vi "LoopselFFcont.VI"() -> ()   [LabVIEW 2015]
panel:
  in  "?":enum32{"1", "2", "3"}(radio)=enum."3"
  in  "pos slope":u8=1
  in  "both slopes":u8
  in  "DAT in 10ns":u32
  out "FIFO overflow":bool
  in  "extTrig 0/1":u8
  in  "stop all":bool
  in  "Slide":u32(slide)=43 scale=1.0..100.0
  in  "frequency[Hz]":u32
  in  "no.of samples (nos)":u32=100
  in  "exposuretime[ms]":dbl=1.0 format="%.3f"
  out "Signalverlaufgraph":u16[](graph)=[4076, 4076, 4076, 4076, 49152, 0, 42, 0, 5277, 5276, 5280, 5289, 5299, 5320, 5298, 5313, 5292, 5320, 5318, 5328, 5333, 5340, 5328, 5331, 5343, 5348, 5338, 5328, 5328, 5329, 5336, 5335, 5343, 5341, 5341, 5331, 5348, 5353, 5349, 5352, 5361, 5365, 5360, 5360, 5367, 5365, 5362, 5372, 5378, 5366, 5379, 5376, 5365, 5378, 5379, 5391, 5376, 5374, 5392, 5411, 5401, 5385, 5382, 5389, 5397, 5390, 5364, 5369, 5381, 5387, 5391, 5387, 5376, 5398, 5395, 5387, 5382, 5377, 5391, 5398, 5407, 5399, 5401, 5418, 5398, 5400, 5391, 5404, 5396, 5394, 5397, 5401, 5390, 5402, 5392, 5394, 5393, 5388, 5389, 5398, 5391, 5377, 5375, 5369, 5388, 5357, 5365, 5359, 5339, 5362, 5354, 5366, 5361, 5352, 5356, 5360, 5352, 5361, 5380, 5378, 5373, 5373, 5365, 5374, 5354, 5364, 5360, 5369, 5367, 5378, 5367, 5382, 5379, 5375, 5378, 5378, 5370, 5369, 5369, 5356, 5359, 5383, 5364, 5356, 5342, 5368, 5376, 5359, 5360, 5367, 5363, 5361, 5379, 5390, 5374, 5346, 5368, 5351, 5390, 5373, 5387, 5363, 5350, 5351, 5347, 5345, 5334, 5331, 5350, 5320, 5328, 5341, 5326, 5327, 5342, 5334, 5340, 5335, 5338, 5335, 5343, 5340, 5337, 5359, 5339, 5331, 5336, 5360, 5345, 5329, 5333, 5327, 5332, 5330, 5309, 5327, 5328, 5332, 5342, 5313, 5304, 5334, 5322, 5319, 5315, 5297, 5310, 5310, 5310, 5293, 5295, 5311, 5285, 5296, 5281, 5297, 5277, 5279, 5293, 5288, 5281, 5286, 5278, 5275, 5273, 5289, 5286, 5283, 5297, 5266, 5268, 5273, 5283, 5269, 5278, 5270, 5268, 5276, 5274, 5272, 5259, 5279, 5263, 5268, 5244, 5265, 5278, 5267, 5259, 5252, 5265, 5266, 5246, 5255, 5257, 5252, 5259, 5274, 5268, 5292, 5296, 5291, 5292, 5292, 5310, 5310, 5324, 5316, 5321, 5344, 5332, 5325, 5305, 5339, 5336, 5340, 5329, 5337, 5345, 5341, 5354, 5368, 5352, 5334, 5347, 5344, 5372, 5364, 5377, 5385, 5370, 5350, 5380, 5375, 5378, 5362, 5379, 5359, 5363, 5365, 5363, 5365, 5357, 5354, 5358, 5342, 5371, 5380, 5370, 5382, 5376, 5399, 5377, 5365, 5370, 5386, 5389, 5360, 5380, 5387, 5364, 5379, 5363, 5363, 5382, 5378, 5390, 5364, 5347, 5386, 5379, 5372, 5361, 5371, 5386, 5386, 5402, 5393, 5402, 5415, 5400, 5411, 5393, 5410, 5402, 5403, 5408, 5412, 5402, 5394, 5396, 5388, 5381, 5387, 5407, 5378, 5384, 5369, 5393, 5386, 5397, 5394, 5393, 5377, 5392, 5391, 5406, 5397, 5389, 5395, 5387, 5391, 5379, 5384, 5397, 5412, 5397, 5395, 5393, 5388, 5368, 5391, 5392, 5391, 5401, 5399, 5396, 5407, 5407, 5395, 5392, 5392, 5433, 5425, 5438, 5441, 5446, 5473, 5438, 5453, 5424, 5444, 5449, 5459, 5448, 5468, 5474, 5465, 5488, 5502, 5495, 5473, 5482, 5483, 5500, 5503, 5509, 5508, 5502, 5496, 5520, 5515, 5518, 5521, 5517, 5515, 5534, 5527, 5538, 5546, 5539, 5543, 5546, 5543, 5572, 5561, 5569, 5565, 5563, 5590, 5572, 5574, 5561, 5583, 5582, 5555, 5556, 5559, 5547, 5558, 5543, 5542, 5558, 5560, 5581, 5561, 5558, 5571, 5565, 5561, 5564, 5554, 5572, 5585, 5590, 5579, 5597, 5609, 5602, 5601, 5606, 5627, 5597, 5630, 5632, 5640, 5622, 5635, 5634, 5641, 5632, 5622, 5640, 5637, 5624, 5586, 5615, 5619, 5629, 5611, 5612, 5595, 5603, 5614, 5615, 5613, 5608, 5624, 5626, 5642, 5635, 5653, 5677, 5682, 5697, 5701, 5696, 5712, 5691, 5709, 5699, 5708, 5725, 5733, 5722, 5737, 5734, 5716, 5723, 5723, 5737, 5730, 5731, 5736, 5752, 5763, 5751, 5762, 5722, 5747, 5753, 5752, 5761, 5766, 5764, 5767, 5778, 5808, 5801, 5781, 5795, 5789, 5812, 5816, 5834, 5823, 5815, 5817, 5848, 5831, 5831, 5827, 5848, 5827, 5840, 5831, 5852, 5852, 5850, 5840, 5842, 5845, 5867, 5858, 5848, 5840, 5851, 5866, 5834, 5847, 5847, 5884, 5865, 5841, 5855, 5847, 5857, 5850, 5844, 5843, 5867, 5848, 5871, 5849, 5845, 5873, 5860, 5844, 5845, 5838, 5852, 5846, 5853, 5841, 5861, 5862, 5859, 5847, 5825, 5845, 5821, 5813, 5807, 5814, 5793, 5801, 5775, 5768, 5752, 5755, 5778, 5751, 5756, 5726, 5745, 5747, 5760, 5742, 5755, 5727, 5712, 5745, 5731, 5726, 5704, 5715, 5707, 5712, 5697, 5688, 5697, 5705, 5707, 5685, 5681, 5685, 5664, 5685, 5674, 5683, 5676, 5684, 5670, 5687, 5680, 5704, 5678, 5678, 5660, 5673, 5685, 5664, 5684, 5718, 5688, 5685, 5682, 5716, 5712, 5713, 5733, 5734, 5731, 5736, 5750, 5765, 5760, 5754, 5768, 5761, 5794, 5804, 5808, 5817, 5813, 5797, 5829, 5806, 5809, 5824, 5835, 5823, 5833, 5821, 5843, 5845, 5848, 5847, 5846, 5828, 5855, 5847, 5860, 5860, 5858, 5861, 5847, 5847, 5841, 5865, 5876, 5844, 5852, 5873, 5879, 5888, 5869, 5884, 5895, 5908, 5918, 5915, 5886, 5942, 5943, 5932, 5935, 5932, 5977, 5963, 5976, 5979, 5979, 5999, 5986, 6002, 6013, 6019, 6011, 6022, 6029, 6053, 6040, 6062, 6043, 6065, 6060, 6070, 6095, 6094, 6091, 6075, 6091, 6109, 6134, 6116, 6119, 6126, 6145, 6168, 6166, 6189, 6187, 6202, 6192, 6203, 6201, 6197, 6236, 6232, 6250, 6238, 6240, 6258, 6248, 6298, 6256, 6278, 6284, 6321, 6320, 6347, 6357, 6341, 6345, 6345, 6484, 6493, 6520, 6543, 6543, 6596, 6575, 6598, 6565, 6617, 6650, 6652, 6654, 6659, 6702, 6704, 6716, 6734, 6744, 6707, 6760, 6758, 6785, 6797, 6825, 6851, 6833, 6859, 6862, 6902, 6909, 6930, 6946, 6957, 6966, 7001, 7009, 7030, 7060, 7051, 7095, 7116, 7137, 7180, 7173, 7176, 7226, 7247, 7272, 7282, 7297, 7337, 7352, 7357, 7385, 7400, 7423, 7458, 7457, 7494, 7517, 7522, 7573, 7573, 7598, 7628, 7654, 7677, 7699, 7709, 7743, 7781, 7792, 7806, 7833, 7861, 7890, 7918, 7938, 7975, 8007, 8039, 8071, 8201, 8343, 8472, 8545, 8684, 8781, 8900, 9041, 9174, 9328, 9463, 9699, 9865, 9976, 10092, 10188, 10266, 10363, 10476, 10562, 10647, 10724, 10818, 10899, 10992, 11048, 11133, 11209, 11299, 11364, 11432, 11512, 11636, 11765, 11921, 12014, 11754, 12235, 12262, 12168, 12214, 12077, 12308, 11568, 11568, 12560, 12073, 12414, 11719, 12059, 12077, 12213, 12350, 12026, 12183, 11918, 11864, 12055, 12342, 12128, 11867, 12416, 12025, 12192, 11997, 12278, 11898, 12191, 12431, 12115, 12141, 11903, 12153, 12110, 11801, 12437, 12528, 12423, 11932, 12627, 12345, 12149, 12615, 12257, 12116, 12293, 11953, 12603, 12261, 12666, 12662, 12225, 12318, 12508, 12002, 12565, 12622, 12199, 12454, 12372, 12103, 12123, 12331, 12088, 12322, 12482, 12010, 12523, 12404, 12269, 12063, 12353, 11857, 12358, 12007, 12339, 12372, 12229, 12499, 12305, 12533, 12477, 12282, 11918, 12526, 12075, 12314, 12043, 12445, 11842, 12154, 11837, 12170, 13169, 12522, 13214, 12892, 12475, 12217, 12608, 12192, 12477, 12321, 12296, 12480, 12396, 12554, 12225, 12268, 12325, 11818, 12342, 12080, 12362, 12168, 12424, 11750, 12150, 12974, 12289, 12219, 12437, 12227, 12272, 12068, 12123, 11755, 12117, 11840, 11624, 12420, 12486, 12486, 4083, 4084, 4104, 4092, 4088, 4082, 4083, 4082, 4086, 4086, 4081, 4096, 4095, 4082, 4084, 4086, 4081, 4088, 4067, 4081, 4078, 4080, 4088, 4088, 4086, 4080, 4092, 4080, 4078, 4082, 4082, 4082, 4097, 4099, 4099, 4093, 4079, 4092, 4082, 4087, 4086, 4088, 4091, 4085, 4088, 4084, 4086, 4091, 4091, 4079, 4078, 4090, 4095, 4095, 4095, 4095]
  # "Start with run"
  # "Abort with ESC"
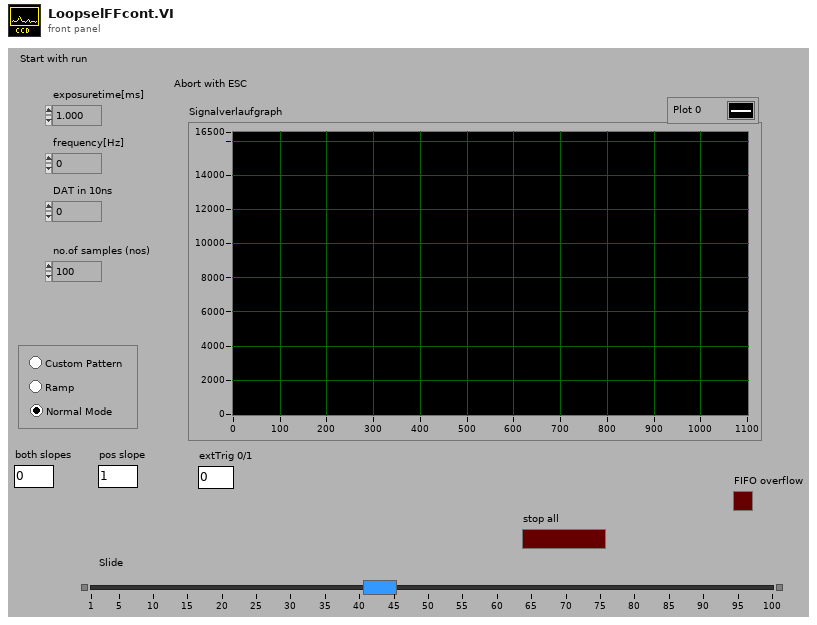
[diagram p1: front panel]
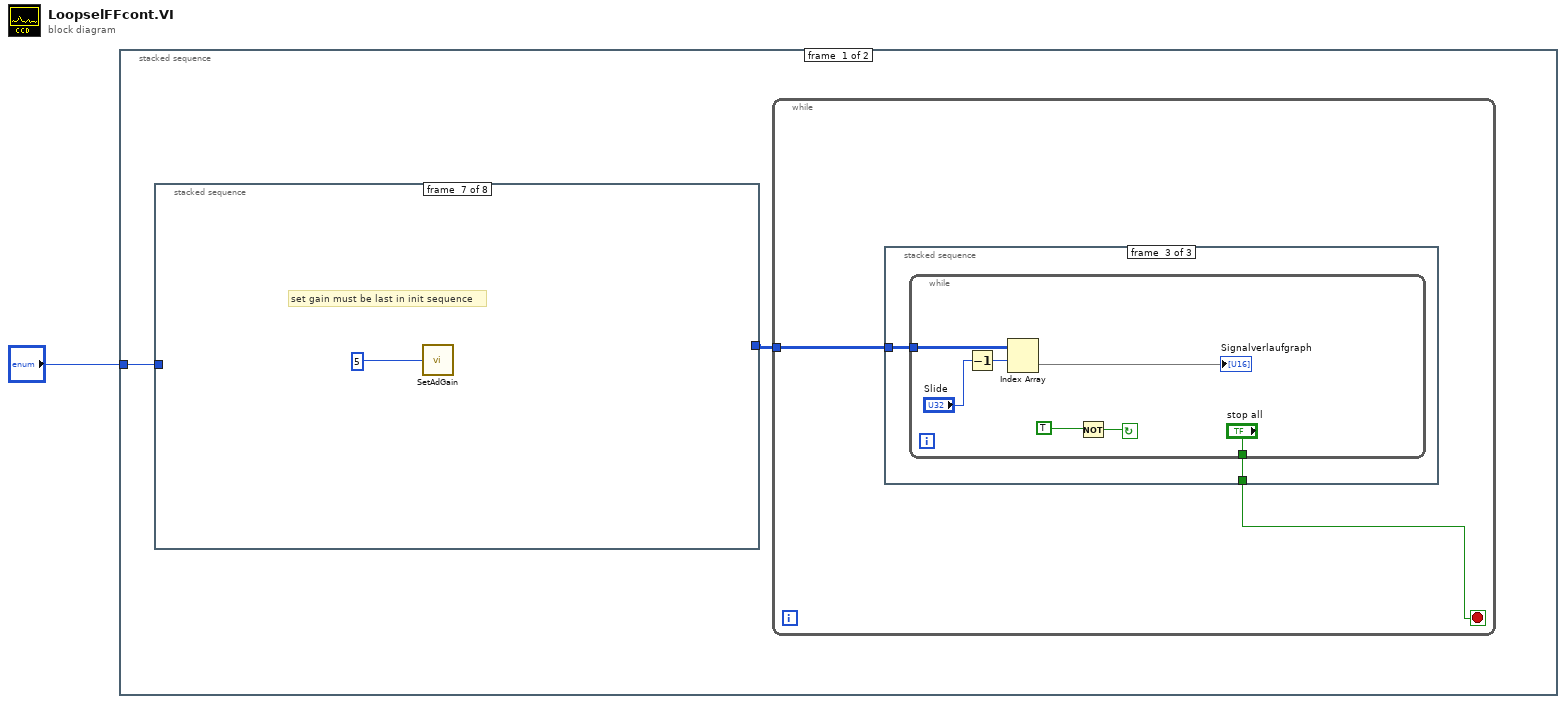
[diagram p0: block diagram]
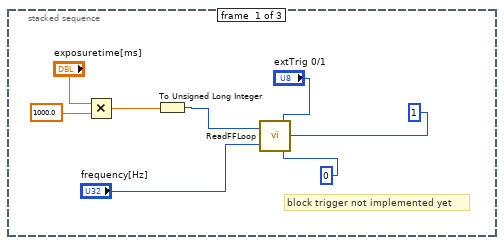
[diagram p2: hidden frame]
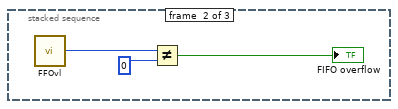
[diagram p3: hidden frame]
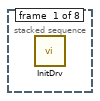
[diagram p4: hidden frame]
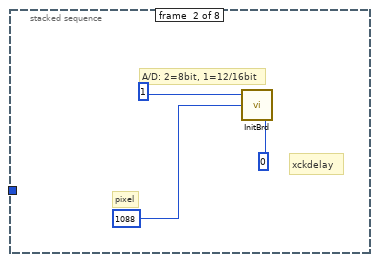
[diagram p5: hidden frame]
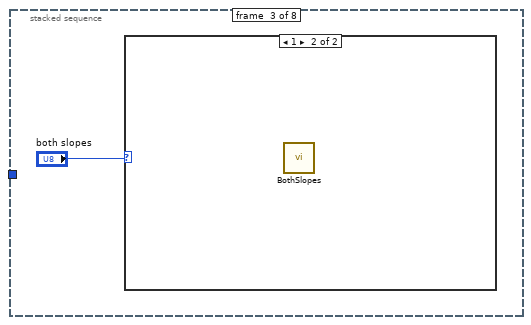
[diagram p6: hidden frame]
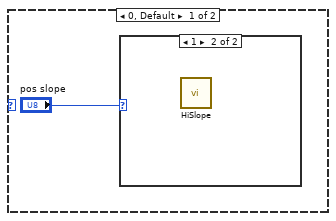
[diagram p7: hidden frame]
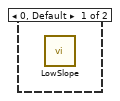
[diagram p8: hidden frame]
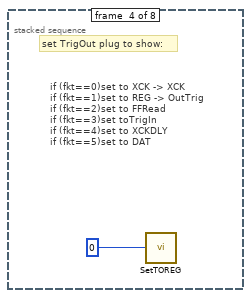
[diagram p9: hidden frame]
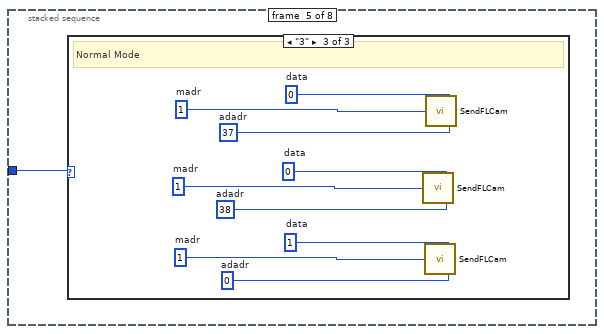
[diagram p10: hidden frame]
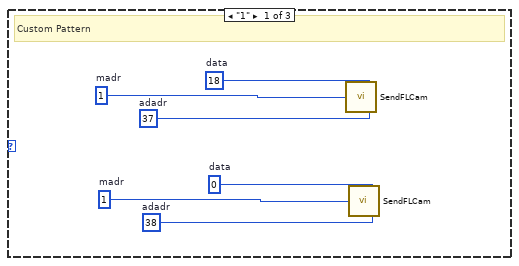
[diagram p11: hidden frame]
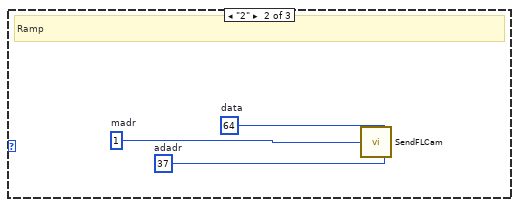
[diagram p12: hidden frame]
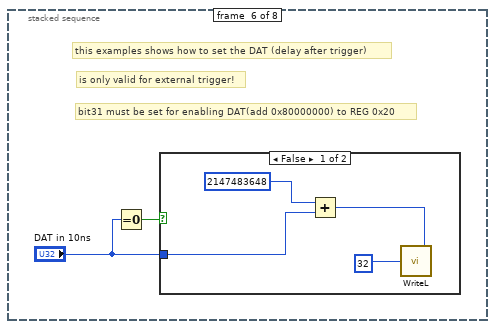
[diagram p13: hidden frame]
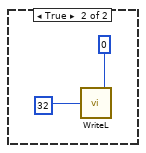
[diagram p14: hidden frame]
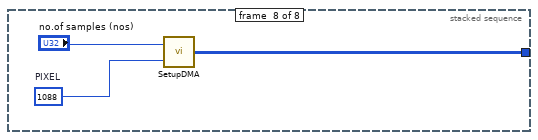
[diagram p15: hidden frame]
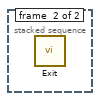
[diagram p16: hidden frame]
diagram:
  n1 = stacked-sequence {
    tunnel: "?" -> [w2 _]
    frame #0 {
      n2 = stacked-sequence {
        tunnel: [_ _ _ _ _ _ _ w62] -> w3
        tunnel: w2 -> [_ _ _ _ w32 _ _ _]
        frame #0 {
          n3 = call "InitDrv.vi"() -> ()  [unwired: 1 in]
        }
        frame #1 {
          # "pixel"
          # "xckdelay"
          # "A/D: 2=8bit, 1=12/16bit"
          n4 = call "InitBrd.vi"("xckdly"=u32 0, "pixel"=u32 1088, "flag816"=u32 1) -> ()  [unwired: 3 in]
        }
        frame #2 {
          n5 = case shown="1" "both slopes" {
            frame 0, Default {
              n6 = case shown="1" "pos slope" {
                frame 0, Default {
                  n7 = call "LowSlope.vi"() -> ()  [unwired: 1 in]
                }
                frame 1 {
                  n8 = call "HiSlope.vi"() -> ()  [unwired: 1 in]
                }
              }
            }
            frame 1 {
              n9 = call "BothSlopes.vi"() -> ()  [unwired: 1 in]
            }
          }
        }
        frame #3 {
          # "set TrigOut plug to show:"
          # "if (fkt==0)set to XCK -> XCK\nif (fkt==1)set to REG -> OutTrig\nif (fkt==2)set to FFRead\nif (fkt==3)set toTrigIn\nif (fkt==4)set to XCKDLY\nif (fkt==5)set to DAT"
          n10 = call "SetTOREG.vi"("fkt"=u8 0) -> ()
        }
        frame #4 {
          n11 = case shown="\"3\"" w32 {
            frame "1" {
              w33 = 0  # data
              w34 = 38  # adadr
              w35 = 1  # madr
              w36 = 18  # data
              w37 = 37  # adadr
              w38 = 1  # madr
              # "Custom Pattern"
              n12 = call "SendFLCam.vi"("madr"=w38, "data"=w36, "adadr"=w37) -> ()
              n13 = call "SendFLCam.vi"("madr"=w35, "data"=w33, "adadr"=w34) -> ()
            }
            frame "2" {
              w39 = 64  # data
              w40 = 37  # adadr
              w41 = 1  # madr
              # "Ramp"
              n14 = call "SendFLCam.vi"("madr"=w41, "data"=w39, "adadr"=w40) -> ()
            }
            frame "3" {
              w42 = 1  # data
              w44 = 0  # adadr
              w43 = 1  # madr
              w47 = 0  # data
              w46 = 38  # adadr
              w45 = 1  # madr
              w50 = 0  # data
              w49 = 37  # adadr
              w48 = 1  # madr
              # "Normal Mode"
              n15 = call "SendFLCam.vi"("madr"=w45, "data"=w47, "adadr"=w46) -> ()
              n16 = call "SendFLCam.vi"("madr"=w43, "data"=w42, "adadr"=w44) -> ()
              n17 = call "SendFLCam.vi"("madr"=w48, "data"=w50, "adadr"=w49) -> ()
            }
          }
        }
        frame #5 {
          # "bit31 must be set for enabling DAT(add 0x80000000) to REG 0x20"
          # "is only valid for external trigger!"
          # "this examples shows how to set the DAT (delay after trigger)"
          n18 = Equal To 0?(x="DAT in 10ns") -> (x = 0?=w52:bool)
          n19 = case shown="False" w52 {
            tunnel: "DAT in 10ns" -> [w53 _]
            frame False {
              n20 = Add(x=u32 2147483648, y=w53) -> (x+y=w56:u32)
              n21 = call "WriteL.vi"("val"=w56, "offset"=u32 32) -> ()
            }
            frame True {
              n22 = call "WriteL.vi"("val"=0, "offset"=u32 32) -> ()
            }
          }
        }
        frame #6 {
          # "set gain must be last in init sequence"
          n23 = call "SetAdGain.vi"("gain"=u8 5) -> ()  [unwired: 1 in]
        }
        frame #7 {
          w61 = u32 1088  # PIXEL
          n24 = call "SetupDMA.vi"("pixel"=w61, "nos"="no.of samples (nos)") -> ("Data Values"=w62:u16[][])
        }
      }
      n25 = while {
        tunnel: w3 -> [w5]
        stop <- w4 stop-if-true
        n26 = stacked-sequence {
          tunnel: w5 -> [_ _ w18]
          tunnel: [_ _ w17] -> w4
          frame #0 {
            # "block trigger not implemented yet"
            n27 = Multiply(x="exposuretime[ms]", y=1000.0) -> (x*y=w13:dbl)
            n28 = To Unsigned Long Integer(number=w13) -> (unsigned 32bit integer=w10:u32)
            n29 = call "ReadFFLoop.vi"("exptus"=w10, "freq"="frequency[Hz]", "ExtTrig"="extTrig 0/1", "btrig_ch"=u32 1, "blocktrigger"=u8 0) -> ()
          }
          frame #1 {
            n30 = call "FFOvl.vi"() -> ("FFOvl"=w15:u8)  [unwired: 1 in]
            n31 = Not Equal?(x=w15, y=0) -> (x != y?=→"FIFO overflow":bool)
          }
          frame #2 {
            n32 = while {
              tunnel: w18 -> [w22]
              tunnel: ["stop all"] -> w17
              stop <- w25 continue-if-true
              n33 = Decrement(x="Slide") -> (x-1=w24:u32)
              n34 = Index Array(array=w22, index (row)=w24) -> (element=→"Signalverlaufgraph":u16[])  [unwired: 1 in]
              n35 = Not(x=TRUE) -> (.not. x?=w25:bool)
            }
          }
        }
      }
    }
    frame #1 {
      n36 = call "Exit.vi"() -> ()  [unwired: 1 in]
    }
  }
